vi "Performance Tests.vi"() -> ()   [LabVIEW 2019]
panel:
  out "XY Graph 2":cluster{i32[], dbl[]}[](graph)
  out "XY Graph 3":cluster{i32[], u32[]}[](graph)
  out "XY Graph":cluster{i32[], u32[]}[](graph)
  in  "Path":path=path "C:/user/patrick/git/LV-to-ITX/src/Tests/Test Files"
  # "DAT"
  # "ITX"
  # "TDMS"
  # "HDF5"
  # "VI"
  # "DAT"
  # "ITX"
  # "TDMS"
  # "HDF5"
  # "VI"
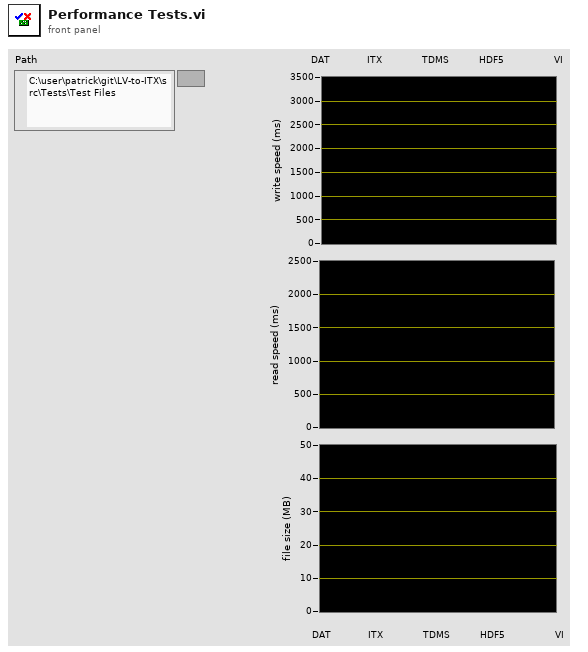
[diagram p1: front panel]
types:
  T1 = cluster{"DAT size (in bytes)":i64, "ITX size (in bytes)":i64, "TDMS size (in bytes)":i64, "HDF5 size (in bytes)":i64, "VI size (in bytes)":i64}
  T2 = cluster{"Write DAT (ms)":u32, "Write ITX (ms)":u32, "Write TDMS (ms)":u32, "Write HDF5 (ms)":u32, "Write VI (ms)":u32}
  T3 = cluster{"Read DAT (ms)":u32, "Read ITX (ms)":u32, "Read TDMS (ms)":u32, "Read HDF5 (ms)":u32, "Read VI (ms)":u32}
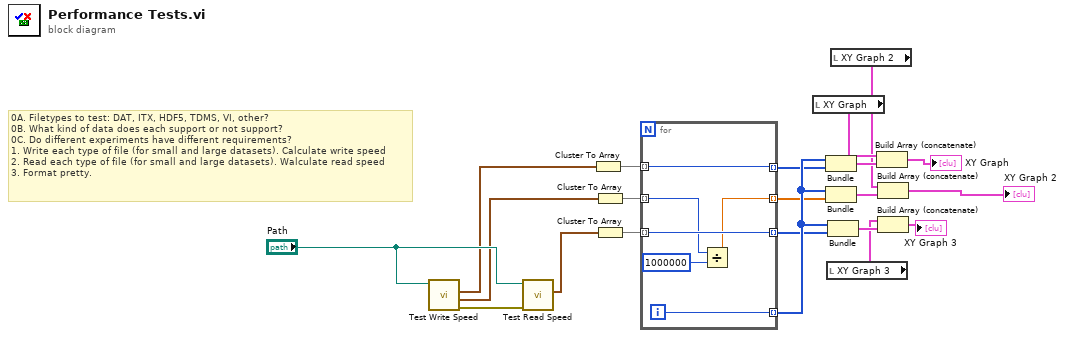
[diagram p0: block diagram]
diagram:
  # "0A. Filetypes to test: DAT, ITX, HDF5, TDMS, VI, other?\n0B. What kind of data does each support or not support?\n0C. Do different experiments have different requirements?\n1. Write each type of file (for small and large datasets). Calculate write speed\n2. Read each type of file (for small and large datasets). Walculate read speed\n3. Format pretty."
  n1 = call "Test Write Speed.vi"("Path"="Path") -> ("error out"=w21:errorcluster, "sizes"=w18:T1, "Write Times"=w19:T2)  [unwired: 8 in]
  n2 = call "Test Read Speed.vi"("error in (no error)"=w21, "Path"="Path") -> ("Read Times"=w17:T3)  [unwired: 8 in, 1 out]
  n3 = Cluster To Array(cluster=w19) -> (array=w16:u32[])
  n4 = Cluster To Array(cluster=w18) -> (array=w15:i64[])
  n5 = Cluster To Array(cluster=w17) -> (array=w14:u32[])
  n6 = for {
    tunnel: w16 -> [w25] mode=indexing
    tunnel: w15 -> [w23] mode=indexing
    tunnel: w14 -> [w24] mode=indexing
    tunnel: [w25] -> w11 mode=indexing
    tunnel: [w22] -> w12 mode=indexing
    tunnel: [w26] -> w13 mode=indexing
    tunnel: [w24] -> w10 mode=indexing
    i -> [w26]
    n7 = Divide(x=w23, y=i64 1000000) -> (x/y=w22:dbl)
  }
  n8 = local read "XY Graph"() -> (w3:cluster{i32[], u32[]}[])
  n9 = Bundle(w13, w11) -> (w9:cluster{i32[], u32[]})  [unwired: 1 in]
  n10 = Bundle(w13, w12) -> (w7:cluster{i32[], dbl[]})  [unwired: 1 in]
  n11 = local read "XY Graph 3"() -> (w1:cluster{i32[], u32[]}[])
  n12 = Bundle(w13, w10) -> (w6:cluster{i32[], u32[]})  [unwired: 1 in]
  n13 = local read "XY Graph 2"() -> (w2:cluster{i32[], dbl[]}[])
  n14 = Build Array (concatenate)(w3, w9) -> (→"XY Graph":cluster{i32[], u32[]}[])
  n15 = Build Array (concatenate)(w2, w7) -> (→"XY Graph 2":cluster{i32[], dbl[]}[])
  n16 = Build Array (concatenate)(w1, w6) -> (→"XY Graph 3":cluster{i32[], u32[]}[])
